vi "Get Bus_Monitor_API StreamBus Request.vi"(8 "error in (no error)":errorcluster, 11 "gRPCid":T1) -> (0 "error out":errorcluster, 2 "Message Data":T2, 3 "gRPCid out":T1)   [LabVIEW 2025, in "bus_monitor_server.lvlib" / "Bus_Monitor_API.lvclass"]
uses:
  Bus_Monitor_API.lvclass
  <vilib>/gRPC/LabVIEW gRPC Library/Shared/grpcId.ctl
  Bus_Monitor_API.lvclass/Bus_Monitor_API.ctl
  bus_monitor_server.lvlib
  <vilib>/gRPC/LabVIEW gRPC Library/grpc-lvsupport-release.lvlib
  RPC Messages/ni_bus_monitor_api_Session.ctl
  RPC Messages/ni_bus_monitor_api_StreamBusRequest.ctl
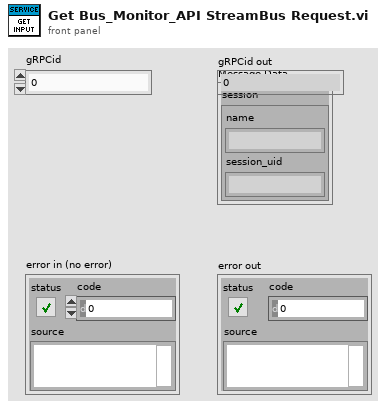
[diagram p1: front panel]
types:
  T1 = typedef "grpc-lvsupport-release.lvlib/grpcId.ctl" = u64
  T2 = typedef "bus_monitor_server.lvlib/ni_bus_monitor_api_StreamBusRequest.ctl" = cluster{"session":T3}
  T3 = typedef "bus_monitor_server.lvlib/ni_bus_monitor_api_Session.ctl" = cluster{"name":string, "session_uid":string}
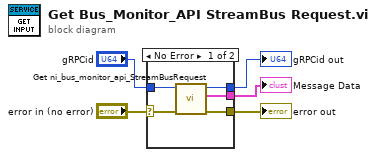
[diagram p0: block diagram]
diagram:
  n1 = case shown="No Error" "error in (no error)" {
    selector: "error in (no error)" -> [w10 w12]
    tunnel: [w9 w12] -> w4
    tunnel: [w8 _] -> w3
    tunnel: "gRPCid" -> [w7 w11]
    tunnel: [w6 w11] -> w1
    frame No Error {
      n2 = call "Get ni_bus_monitor_api_StreamBusRequest.vi"("error in (no error)"=w10, "gRPCid"=w7) -> ("error out"=w9:errorcluster, "package_templatemessage"=w8:T2, "gRPCid out"=w6:T1)  [unwired: 7 in]
    }
    frame Error {
    }
  }
  "error out" <- w4
  "Message Data" <- w3
  "gRPCid out" <- w1
